vi "Test animation.vi"(8 "error in (no error)":errorcluster, 10 "Hide?":bool=TRUE, 11 "Counts cluster":refnum<vi>) -> (0 "error out":errorcluster)   [LabVIEW 2019]
uses:
  <vilib>/Utility/miscctls.llb/LVBoundsTypeDef.ctl
panel:
  out "Current position":i32
  out "Bounds":T1
  out "Current position FAIL":i32
  out "Current position PASS":i32
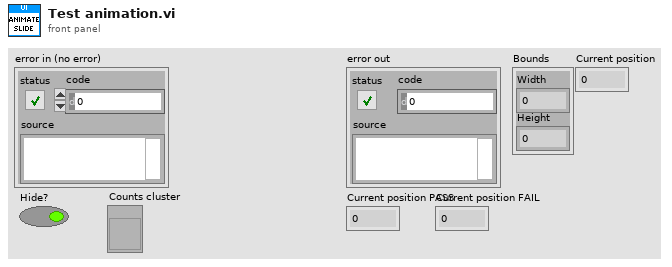
[diagram p1: front panel]
types:
  T1 = typedef "LVBoundsTypeDef.ctl" = cluster{"Width":u32, "Height":u32}
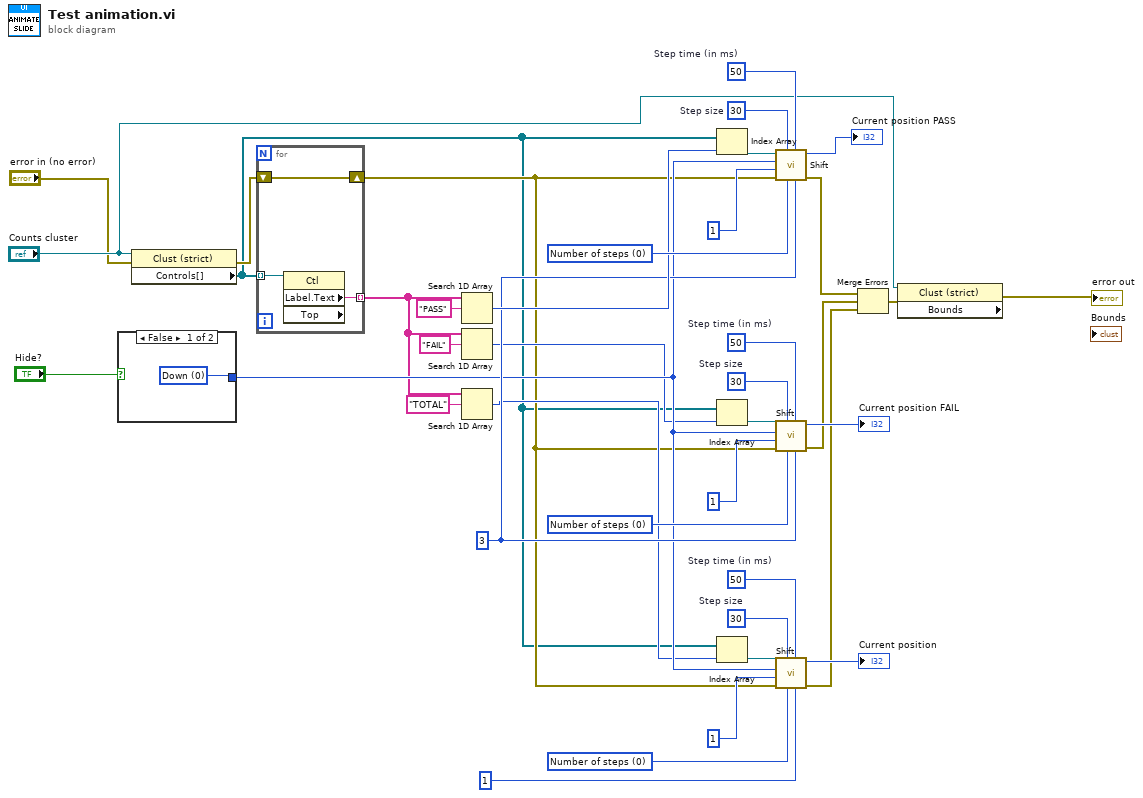
[diagram p0: block diagram]
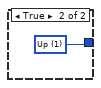
[diagram p2: hidden frame]
diagram:
  w15 = u16 0 items=["Number of steps", "Absolute position"] ("Absolute position")
  w16 = u32 50  # Step time (in ms)
  w17 = 30  # Step size
  w20 = 3 ("Step count")
  w30 = u16 0 items=["Number of steps", "Absolute position"] ("Absolute position")
  w29 = u32 50  # Step time (in ms)
  w28 = 30  # Step size
  w32 = u16 0 items=["Number of steps", "Absolute position"] ("Absolute position")
  w34 = u32 50  # Step time (in ms)
  w35 = 30  # Step size
  n1 = case shown="False" "Hide?" {
    tunnel: [w40 w41] -> w14
    frame False {
      w40 = u16 0 items=["Down", "Up", "Right", "Left"] ("Hide / Unhide?")
    }
    frame True {
      w41 = u16 1 items=["Down", "Up", "Right", "Left"] ("Hide / Unhide?")
    }
  }
  n2 = property class="Clust (strict)"(reference="Counts cluster", error in="error in (no error)") -> (error out=w3:errorcluster, "Controls[]"=w1:refnum<vi>[])  [unwired: 1 out]
  n3 = for {
    tunnel: w1 -> [w44] mode=indexing
    tunnel: [w43] -> w11 mode=indexing
    shift-right: [w42] -> w2
    shift-left: w3 -> [w42]
    n4 = property class="Ctl" props=["Label", "Text", "Top"](reference=w44) -> ("Label.Text"=w43:string)  [unwired: 1 in, 3 out]
  }
  n5 = Search 1D Array(1D array=w11, element="PASS") -> (index of element=w31:i32)  [unwired: 1 in]
  n6 = Search 1D Array(1D array=w11, element="FAIL") -> (index of element=w13:i32)  [unwired: 1 in]
  n7 = Search 1D Array(1D array=w11, element="TOTAL") -> (index of element=w9:i32)  [unwired: 1 in]
  n8 = Index Array(array=w1, index=w31) -> (element=w37:refnum<vi>)
  n9 = Index Array(array=w1, index=w13) -> (element=w26:refnum<vi>)
  n10 = Index Array(array=w1, index=w9) -> (element=w19:refnum<vi>)
  n11 = call "Shift.vi"("Step count"=w20, "Step time (in ms)"=w34, "Absolute position"=w32, "Step size"=w35, "error in (no error)"=w2, "Final position"=1, "Movement direction"=w14, "Control in"=w37) -> ("error out"=w24:errorcluster, "Current position"=→"Current position PASS":i32)  [unwired: 2 in]
  n12 = call "Shift.vi"("Step count"=w20, "Step time (in ms)"=w29, "Absolute position"=w30, "Step size"=w28, "error in (no error)"=w2, "Final position"=1, "Movement direction"=w14, "Control in"=w26) -> ("error out"=w23:errorcluster, "Current position"=→"Current position FAIL":i32)  [unwired: 2 in]
  n13 = call "Shift.vi"("Step count"=1, "Step time (in ms)"=w16, "Absolute position"=w15, "Step size"=w17, "error in (no error)"=w2, "Final position"=1, "Movement direction"=w14, "Control in"=w19) -> ("error out"=w7:errorcluster, "Current position"=→"Current position":i32)  [unwired: 2 in]
  n14 = Merge Errors(w24, w23, w7) -> (w22:errorcluster)
  n15 = property class="Clust (strict)" props=["Bounds"](reference="Counts cluster", error in=w22) -> (error out=→"error out":errorcluster)  [unwired: 2 out]
